vi "CheckFileOverwrite.vi"(9 "Code in":string, 10 "Tree":string, 11 "OldVal":string) -> (3 "Code out":string)   [LabVIEW 2020]
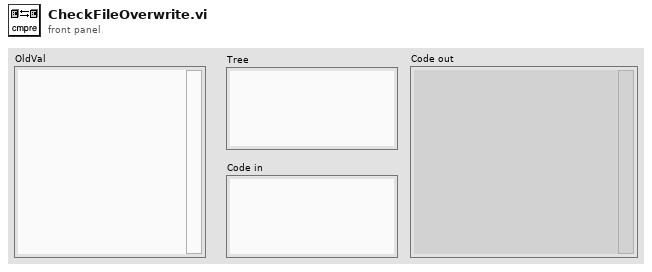
[diagram p1: front panel]
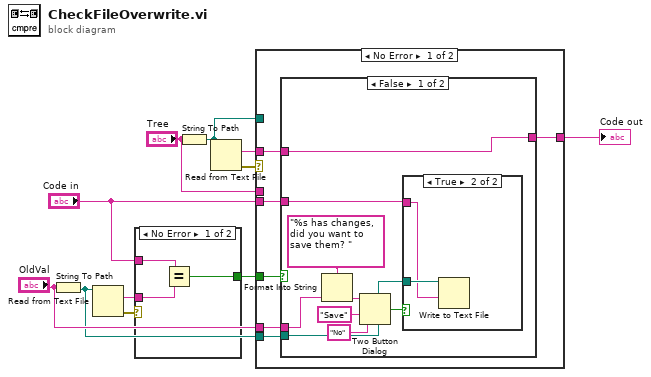
[diagram p0: block diagram]
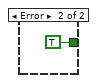
[diagram p2: hidden frame]
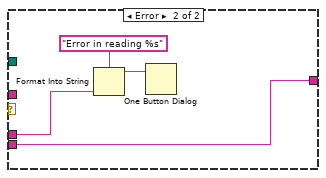
[diagram p5: hidden frame]
diagram:
  n1 = String To Path(string="OldVal") -> (path=w2:path)
  n2 = Read from Text File(file (use dialog)=w2) -> (text=w1:string, error out=w6:errorcluster)  [unwired: 3 in, 2 out]
  n3 = case shown="No Error" w6 {
    tunnel: w1 -> [w12 _]
    tunnel: "Code in" -> [w14 _]
    tunnel: [w13 TRUE] -> w4
    frame No Error {
      n4 = Equal?(x=w14, y=w12) -> (x = y?=w13:bool)
    }
    frame Error {
    }
  }
  n5 = String To Path(string="Tree") -> (path=w8:path)
  n6 = Read from Text File(file (use dialog)=w8) -> (text=w11:string, error out=w7:errorcluster)  [unwired: 3 in, 2 out]
  n7 = case shown="No Error" w7 {
    tunnel: w8 -> [_ _]
    tunnel: "Tree" -> [_ w35]
    tunnel: [w20 w34] -> w10
    tunnel: w11 -> [w19 _]
    tunnel: "Code in" -> [w16 w34]
    tunnel: w4 -> [w21 _]
    tunnel: "OldVal" -> [w18 _]
    tunnel: w2 -> [w17 _]
    frame No Error {
      n8 = case shown="False" w21 {
        tunnel: [w25 w33] -> w20
        tunnel: w19 -> [w25 w33]
        tunnel: w18 -> [w30 _]
        tunnel: w17 -> [w26 _]
        tunnel: w16 -> [w22 _]
        frame False {
          n9 = Format Into String(format string="%s has changes, did you want to save them? " ("message"), w30) -> (resulting string=w28:string)  [unwired: 2 in, 1 out]
          n10 = Two Button Dialog(message=w28, 1:"No" ("F button name (\"Cancel\")"), 2:"Save" ("T button name (\"OK\")")) -> (T button?=w27:bool)
          n11 = case shown="True" w27 {
            tunnel: w26 -> [_ w32]
            tunnel: w22 -> [_ w31]
            frame False {
            }
            frame True {
              n12 = Write to Text File(file (use dialog)=w32, text=w31) -> ()  [unwired: 2 in, 3 out]
            }
          }
        }
        frame True {
        }
      }
    }
    frame Error {
      n13 = Format Into String(format string="Error in reading %s" ("message"), w35) -> (resulting string=w36:string)  [unwired: 2 in, 1 out]
      n14 = One Button Dialog(message=w36) -> ()  [unwired: 1 in, 1 out]
    }
  }
  "Code out" <- w10
